vi "sub_log-load_ubx.vi"() -> ()   [LabVIEW 2019]
panel:
  in  "sel file - str":bool
  out "val":bool
  out "XY 그래프":cluster{"X":dbl, "Y":dbl}[](graph)
  in  "정지":bool
  out "heading imu":dbl[](array[numeric]) format="%01.1f"
  out "이전 부분 문자열":string
  out "heading tracing":dbl[](array[numeric]) format="%01.1f"
  out "latlong out":cluster{"Lat":dbl, "Long":dbl}[](array[cluster])
  out "tm out":cluster{"XE":dbl, "YN":dbl}[](array[cluster])
  out "n":i32=24061
  out "tm graph":cluster{"X":dbl, "Y":dbl}[](graph)=[{"X"=195463.43833256784, "Y"=532664.2368708845}, {"X"=195463.37935875848, "Y"=532664.3478879803}, {"X"=195463.37944915734, "Y"=532664.5143655398}, {"X"=195463.33526400154, "Y"=532664.6808671424}, {"X"=195463.23200460023, "Y"=532664.7734107748}, {"X"=195463.18778931902, "Y"=532664.8844198572}, {"X"=195463.158302417, "Y"=532664.939928406}, {"X"=195463.02545567148, "Y"=532664.9030055237}, {"X"=195462.96640151046, "Y"=532664.8660425695}, {"X"=195462.8335346741, "Y"=532664.7921246769}, {"X"=195462.74496347454, "Y"=532664.7551777533}, {"X"=195462.77457092013, "Y"=532664.9216392826}, {"X"=195463.42418674467, "Y"=532665.3652268056}, {"X"=195464.41330861498, "Y"=532665.9196151308}, {"X"=195465.49103164242, "Y"=532666.5664430471}, {"X"=195466.5393478853, "Y"=532667.4167596921}, {"X"=195467.73517878767, "Y"=532668.1375138587}, {"X"=195469.03423880192, "Y"=532668.7102321138}, {"X"=195470.27427462512, "Y"=532669.3014800847}, {"X"=195471.3814636429, "Y"=532669.8558052257}, {"X"=195472.53304832894, "Y"=532670.6320766001}, {"X"=195473.68450251664, "Y"=532671.1678805449}, {"X"=195474.82121809167, "Y"=532671.7406876583}, {"X"=195475.88423113854, "Y"=532672.4800124469}, {"X"=195476.94724399722, "Y"=532673.219337371}, {"X"=195478.0102466557, "Y"=532673.9401649248}, {"X"=195479.1764785589, "Y"=532674.5129566543}, {"X"=195480.32796180525, "Y"=532675.1042540387}, {"X"=195481.44992789478, "Y"=532675.6955675457}, {"X"=195482.6161893219, "Y"=532676.3238522782}, {"X"=195483.69397958953, "Y"=532677.1001650991}, {"X"=195484.6829887544, "Y"=532677.4510832544}, {"X"=195485.83431129332, "Y"=532677.7464212874}, {"X"=195487.10376165676, "Y"=532678.1526807427}, {"X"=195488.37312199303, "Y"=532678.3924628282}, {"X"=195489.36211083402, "Y"=532678.7063865255}, {"X"=195490.14448070675, "Y"=532679.0204218699}, {"X"=195491.16320601458, "Y"=532679.741275002}, {"X"=195492.19687926685, "Y"=532680.8135729311}, {"X"=195493.03851230364, "Y"=532681.5530193599}, {"X"=195494.1160914222, "Y"=532681.9408858792}, {"X"=195495.26754266868, "Y"=532682.4766928047}, {"X"=195496.15353049224, "Y"=532683.3640957345}, {"X"=195497.29010329436, "Y"=532683.6779408107}, {"X"=195498.39734841217, "Y"=532684.3432545831}, {"X"=195499.41604246455, "Y"=532685.0086162025}, {"X"=195500.8330559466, "Y"=532685.3778032307}, {"X"=195502.2500294698, "Y"=532685.6730004699}, {"X"=195503.38700991592, "Y"=532686.7452441752}, {"X"=195504.67135587469, "Y"=532687.4104634614}, {"X"=195505.88195899536, "Y"=532688.1682101777}, {"X"=195506.95982515637, "Y"=532689.0925060686}, {"X"=195508.05230036922, "Y"=532689.7393315544}, {"X"=195509.3218273631, "Y"=532690.2935744494}, {"X"=195510.63554014615, "Y"=532690.6813161802}, {"X"=195511.99361765472, "Y"=532691.2355118981}, {"X"=195513.08586370462, "Y"=532691.4568953742}, {"X"=195514.2076465018, "Y"=532691.7152581579}, {"X"=195515.32960795384, "Y"=532692.3065762268}, {"X"=195516.46638728245, "Y"=532693.0088715698}, {"X"=195517.58840795147, "Y"=532693.7111749877}, {"X"=195518.78410169733, "Y"=532694.1914688842}, {"X"=195519.99460336298, "Y"=532694.764242577}, {"X"=195521.1460511766, "Y"=532695.3000530777}, {"X"=195522.07599301488, "Y"=532695.5955147923}, {"X"=195523.1535293239, "Y"=532695.9093950319}, {"X"=195524.08341156298, "Y"=532696.0938719255}, {"X"=195524.5705894479, "Y"=532696.3710736269}, {"X"=195524.7034156071, "Y"=532696.3710024743}, {"X"=195524.74775044026, "Y"=532696.4819638014}, {"X"=195524.7478396172, "Y"=532696.6484413707}, {"X"=195524.85116866234, "Y"=532696.685381046}, {"X"=195524.89544404706, "Y"=532696.6853573297}, {"X"=195524.99875327287, "Y"=532696.6853019926}, {"X"=195525.07256539716, "Y"=532696.7222574817}, {"X"=195525.16117560753, "Y"=532696.8331950981}, {"X"=195525.29412064294, "Y"=532697.0550940447}, {"X"=195525.42702604536, "Y"=532697.2030029638}, {"X"=195525.57471962064, "Y"=532697.4063965041}, {"X"=195525.7075655717, "Y"=532697.4433203822}, {"X"=195525.79613614336, "Y"=532697.4802679741}, {"X"=195525.88469680815, "Y"=532697.4987180593}, {"X"=195525.98805555515, "Y"=532697.5911502724}, {"X"=195526.06185775693, "Y"=532697.609608263}, {"X"=195526.13568967706, "Y"=532697.683558776}, {"X"=195526.19477304455, "Y"=532697.776014701}, {"X"=195526.26859505233, "Y"=532697.8314677086}, {"X"=195526.3423873486, "Y"=532697.8314281941}, {"X"=195526.40143109093, "Y"=532697.849894091}, {"X"=195526.460474833, "Y"=532697.8683599874}, {"X"=195526.50474030682, "Y"=532697.8498387724}, {"X"=195526.4308588673, "Y"=532697.6834007172}, {"X"=195526.47517386338, "Y"=532697.7573670406}, {"X"=195526.50470068818, "Y"=532697.7758487416}, {"X"=195526.53420770136, "Y"=532697.7573354304}, {"X"=195526.54897606486, "Y"=532697.7758250341}, {"X"=195526.60804951593, "Y"=532697.8497834553}, {"X"=195526.68190123988, "Y"=532697.9607289893}, {"X"=195526.88855927964, "Y"=532698.0346083909}, {"X"=195526.96240109234, "Y"=532698.1270564198}, {"X"=195527.02141511615, "Y"=532698.0900297988}, {"X"=195527.08041924387, "Y"=532698.0345056687}, {"X"=195527.1247342301, "Y"=532698.108471994}, {"X"=195526.8884206263, "Y"=532697.7756432841}, {"X"=195526.77026381393, "Y"=532697.6092289329}, {"X"=195526.79978073458, "Y"=532697.6092131288}, {"X"=195526.8293570766, "Y"=532697.7201823699}, {"X"=195526.85892351624, "Y"=532697.8126541035}, {"X"=195527.00666656136, "Y"=532698.1085352066}, {"X"=195527.4348500131, "Y"=532698.4597587141}, {"X"=195528.24687212674, "Y"=532699.0327469374}, {"X"=195529.32456613673, "Y"=532699.6425880961}, {"X"=195530.63829630864, "Y"=532700.0673279922}, {"X"=195531.9963610663, "Y"=532700.6030294579}, {"X"=195533.33957819303, "Y"=532700.9722614696}, {"X"=195534.72692225696, "Y"=532701.0640074186}, {"X"=195536.1290939311, "Y"=532701.285228265}, {"X"=195537.44268517097, "Y"=532701.4510041233}, {"X"=195538.7415277862, "Y"=532701.6352855739}, {"X"=195540.0404394645, "Y"=532701.9490497827}, {"X"=195541.3246518252, "Y"=532702.3738071152}, {"X"=195542.65322822542, "Y"=532702.9650185935}, {"X"=195543.92269171606, "Y"=532703.4082817067}, {"X"=195545.19214520394, "Y"=532703.8330475076}, {"X"=195546.55014925377, "Y"=532704.2577662958}, {"X"=195547.87866584174, "Y"=532704.7379935593}, {"X"=195549.28095479903, "Y"=532705.181186705}, {"X"=195550.638899309, "Y"=532705.4949211149}, {"X"=195552.08545347524, "Y"=532705.9195936443}, {"X"=195553.48777154498, "Y"=532706.4182800212}, {"X"=195554.84590269416, "Y"=532707.0834677607}, {"X"=195556.0563803374, "Y"=532707.6192516707}, {"X"=195557.20781422194, "Y"=532708.1365696405}, {"X"=195558.40351345303, "Y"=532708.6353667225}, {"X"=195559.62873925007, "Y"=532709.1526457963}, {"X"=195560.85396489518, "Y"=532709.6699250496}, {"X"=195562.07921003803, "Y"=532710.2241994971}, {"X"=195563.289716231, "Y"=532710.8154769803}, {"X"=195564.54451719543, "Y"=532711.443726148}, {"X"=195565.81412549742, "Y"=532712.1644552109}, {"X"=195566.95081935, "Y"=532712.7187773762}, {"X"=195568.14656640016, "Y"=532713.3100633936}, {"X"=195569.38656895916, "Y"=532713.8643310885}, {"X"=195570.65612743786, "Y"=532714.4925733493}, {"X"=195571.82244535882, "Y"=532715.2503531169}, {"X"=195573.00352149023, "Y"=532716.0081252258}, {"X"=195574.12556370843, "Y"=532716.7659287783}, {"X"=195575.26236414464, "Y"=532717.5237246654}, {"X"=195576.51714361613, "Y"=532718.1149806204}, {"X"=195577.75707636445, "Y"=532718.5397670033}, {"X"=195579.0412646738, "Y"=532718.9275351231}, {"X"=195580.2369512657, "Y"=532719.4078378282}, {"X"=195581.55071486297, "Y"=532719.9065757681}, {"X"=195582.79060796814, "Y"=532720.2573728659}, {"X"=195583.9122771791, "Y"=532720.3122724262}, {"X"=195585.18163808706, "Y"=532720.570566735}, {"X"=195586.51004236046, "Y"=532720.8473275584}, {"X"=195587.80901763373, "Y"=532721.2905817559}, {"X"=195589.0932441141, "Y"=532721.7523414554}, {"X"=195590.28889067026, "Y"=532722.1586555662}, {"X"=195591.52884163495, "Y"=532722.620439012}, {"X"=195592.82786515707, "Y"=532723.1561815299}, {"X"=195594.12691777293, "Y"=532723.7474167764}, {"X"=195595.4554480201, "Y"=532724.264646632}, {"X"=195596.72497370603, "Y"=532724.837400335}, {"X"=195597.92078514092, "Y"=532725.5581731821}, {"X"=195599.1460547227, "Y"=532726.1679456017}, {"X"=195600.4893816471, "Y"=532726.759158516}, {"X"=195601.78835525474, "Y"=532727.2024148892}, {"X"=195603.01357563346, "Y"=532727.7197003352}, {"X"=195604.23879586247, "Y"=532728.2369859603}, {"X"=195605.5083106137, "Y"=532728.791243493}, {"X"=195606.777834921, "Y"=532729.3639987274}, {"X"=195608.06209800762, "Y"=532729.89975138}, {"X"=195609.3463609293, "Y"=532730.4355042303}, {"X"=195610.55678308988, "Y"=532730.8788085075}, {"X"=195611.8262484379, "Y"=532731.3405794604}, {"X"=195613.09573307371, "Y"=532731.8393456227}, {"X"=195614.30626164764, "Y"=532732.4861230355}, {"X"=195615.53155813567, "Y"=532733.1513903878}, {"X"=195616.8010810917, "Y"=532733.7241471487}, {"X"=195618.01163820943, "Y"=532734.4264176253}, {"X"=195619.25173131019, "Y"=532735.1656678186}, {"X"=195620.43281971622, "Y"=532735.9604416658}, {"X"=195621.56966180843, "Y"=532736.8107314138}, {"X"=195622.69168712775, "Y"=532737.5500439969}, {"X"=195623.8432193357, "Y"=532738.270843762}, {"X"=195624.9947416581, "Y"=532738.9731461777}, {"X"=195626.3085188666, "Y"=532739.5088861827}, {"X"=195627.50417074907, "Y"=532739.933703138}, {"X"=195628.75890443352, "Y"=532740.4509769174}, {"X"=195629.82173060603, "Y"=532740.8758637004}, {"X"=195630.91406376034, "Y"=532741.2822376763}, {"X"=195632.2130238219, "Y"=532741.7070012771}, {"X"=195633.55624922222, "Y"=532742.113244432}, {"X"=195635.03243521648, "Y"=532742.778383525}, {"X"=195636.36106617516, "Y"=532743.4990924905}, {"X"=195637.704397334, "Y"=532744.1088089084}, {"X"=195639.18054402331, "Y"=532744.6999587019}, {"X"=195640.62720270804, "Y"=532745.3466166832}, {"X"=195641.95580382948, "Y"=532746.0118340147}, {"X"=195643.31387325283, "Y"=532746.5845486206}, {"X"=195644.73091811733, "Y"=532747.046247619}, {"X"=195646.13317553644, "Y"=532747.4524620217}, {"X"=195647.47639933572, "Y"=532747.8587074166}, {"X"=195648.79020260356, "Y"=532748.4499434888}, {"X"=195650.08920879228, "Y"=532748.9671974168}, {"X"=195651.4619970308, "Y"=532749.4659156284}, {"X"=195652.89390520056, "Y"=532750.1310809287}, {"X"=195654.23720521078, "Y"=532750.6853074832}, {"X"=195655.60998330187, "Y"=532751.165528868}, {"X"=195656.95325412156, "Y"=532751.6642633328}, {"X"=195658.3260222799, "Y"=532752.1259876547}, {"X"=195659.68406075655, "Y"=532752.6432123989}, {"X"=195661.0568189934, "Y"=532753.0864396617}, {"X"=195662.38530200603, "Y"=532753.5296901399}, {"X"=195663.62526352247, "Y"=532754.0284793162}, {"X"=195664.9242295315, "Y"=532754.471745517}, {"X"=195666.41507324539, "Y"=532754.9519074148}, {"X"=195667.81734746048, "Y"=532755.3951204793}, {"X"=195669.1754711147, "Y"=532756.0788243498}, {"X"=195670.47450360752, "Y"=532756.6515739784}, {"X"=195671.7144545975, "Y"=532757.1318668477}, {"X"=195673.01350591303, "Y"=532757.741611891}, {"X"=195674.4453439012, "Y"=532758.2772983258}, {"X"=195675.8181195748, "Y"=532758.757523035}, {"X"=195677.24991892636, "Y"=532759.2192199171}, {"X"=195678.6965147357, "Y"=532759.7548994441}, {"X"=195680.1726461872, "Y"=532760.3275589806}, {"X"=195681.58975361122, "Y"=532760.918746801}, {"X"=195682.9478561166, "Y"=532761.565457895}, {"X"=195684.3059106409, "Y"=532762.1196816645}, {"X"=195685.73775670477, "Y"=532762.673867547}, {"X"=195687.0514976321, "Y"=532763.1541245902}, {"X"=195688.29143715004, "Y"=532763.6159224136}, {"X"=195689.51673271428, "Y"=532764.2996981493}, {"X"=195690.83054950094, "Y"=532764.9279358606}, {"X"=195692.2033899006, "Y"=532765.5376458303}, {"X"=195693.63525392523, "Y"=532766.1288280886}, {"X"=195695.06712727412, "Y"=532766.7385081005}, {"X"=195696.48426113735, "Y"=532767.3851909791}, {"X"=195697.9013566771, "Y"=532767.9578840624}, {"X"=195699.274138932, "Y"=532768.4566101402}, {"X"=195700.6174138786, "Y"=532768.9738491422}, {"X"=195701.84268861313, "Y"=532769.6206316698}, {"X"=195703.20075008267, "Y"=532770.1933560242}, {"X"=195704.4259768832, "Y"=532770.7476513837}, {"X"=195705.66599037888, "Y"=532771.3574318669}, {"X"=195707.0093024787, "Y"=532771.9486619369}, {"X"=195708.36731570578, "Y"=532772.4288995846}, {"X"=195709.65142314986, "Y"=532772.6872052341}, {"X"=195710.89134100443, "Y"=532773.1120113983}, {"X"=195712.21976121952, "Y"=532773.4442847518}, {"X"=195713.66621944733, "Y"=532773.721005208}, {"X"=195715.17156857622, "Y"=532773.720232995}, {"X"=195716.66205505346, "Y"=532773.5159960149}, {"X"=195718.06377359235, "Y"=532772.8863619665}, {"X"=195719.21443964881, "Y"=532771.9423990478}, {"X"=195720.37984534324, "Y"=532770.961433709}, {"X"=195721.42715623864, "Y"=532769.9250364729}, {"X"=195722.2234715443, "Y"=532768.6852952294}, {"X"=195722.81316091242, "Y"=532767.4271623343}, {"X"=195723.37340007036, "Y"=532766.2985271581}, {"X"=195723.8598003337, "Y"=532765.0774422467}, {"X"=195724.36091175413, "Y"=532763.7638622674}, {"X"=195724.96531281195, "Y"=532762.4132344332}, {"X"=195725.55501250137, "Y"=532761.1735992552}, {"X"=195726.14469344265, "Y"=532759.8969691027}, {"X"=195726.6163361366, "Y"=532758.675891914}, {"X"=195727.2504533032, "Y"=532757.7136968506}, {"X"=195727.92869433944, "Y"=532756.4555190526}, {"X"=195728.6955235518, "Y"=532755.2712860733}, {"X"=195729.27039029414, "Y"=532753.8836786455}, {"X"=195729.80093486852, "Y"=532752.403606346}, {"X"=195730.4347787353, "Y"=532750.9049837765}, {"X"=195730.5815966956, "Y"=532749.406610134}, {"X"=195731.171222524, "Y"=532748.0189953073}, {"X"=195731.90859293088, "Y"=532746.9457627758}, {"X"=195732.40967836019, "Y"=532745.5766907893}, {"X"=195732.9550674269, "Y"=532744.2630887484}, {"X"=195733.72191736553, "Y"=532743.1158512731}, {"X"=195734.4001888985, "Y"=532741.9131665553}, {"X"=195735.1226413439, "Y"=532740.5254842079}, {"X"=195735.88943527907, "Y"=532739.2672618876}, {"X"=195736.64145217667, "Y"=532737.9720521529}, {"X"=195737.27547769167, "Y"=532736.8248827985}, {"X"=195738.11613974278, "Y"=532735.7146031067}, {"X"=195738.85340834467, "Y"=532734.4378986182}, {"X"=195739.50221169676, "Y"=532733.3277169282}, {"X"=195740.10667400094, "Y"=532732.0880753087}, {"X"=195740.8586544795, "Y"=532730.7188759372}, {"X"=195741.40409299757, "Y"=532729.49776202}, {"X"=195741.84618512177, "Y"=532728.2027107645}, {"X"=195742.3768749644, "Y"=532727.0001019468}, {"X"=195742.9076215138, "Y"=532725.9084782144}, {"X"=195743.39398929762, "Y"=532724.6134044877}, {"X"=195744.013126419, "Y"=532723.207278077}, {"X"=195744.63225432741, "Y"=532721.7826542063}, {"X"=195745.3547855843, "Y"=532720.5429528507}, {"X"=195746.0919812887, "Y"=532719.118268969}, {"X"=195746.79966039592, "Y"=532717.6936001816}, {"X"=195747.24175398872, "Y"=532716.3985492358}, {"X"=195747.9051864799, "Y"=532715.0293956088}, {"X"=195748.46526311143, "Y"=532713.5678070722}, {"X"=195749.49760981172, "Y"=532712.1059782859}, {"X"=195750.293915986, "Y"=532710.8292448211}, {"X"=195751.04592827562, "Y"=532709.5155389357}, {"X"=195751.7389728836, "Y"=532708.3313456943}, {"X"=195752.29925753924, "Y"=532707.2767025982}, {"X"=195752.71192028275, "Y"=532706.1481445385}, {"X"=195753.25736213874, "Y"=532704.9270314455}, {"X"=195753.92084354223, "Y"=532703.6503658611}, {"X"=195754.30404618176, "Y"=532702.6328079345}, {"X"=195754.48040499454, "Y"=532701.171414843}, {"X"=195754.89309653037, "Y"=532700.0983494235}, {"X"=195755.52714623124, "Y"=532698.9881765428}, {"X"=195755.93978163204, "Y"=532697.8041261351}, {"X"=195756.57385043486, "Y"=532696.7309483497}, {"X"=195757.16371916333, "Y"=532695.8057731603}, {"X"=195757.3255268149, "Y"=532694.751332799}, {"X"=195757.72334785637, "Y"=532693.4563049399}, {"X"=195758.13587114145, "Y"=532692.0502845659}, {"X"=195758.79930736014, "Y"=532690.6811318584}, {"X"=195758.78403241967, "Y"=532689.6637764573}, {"X"=195759.240916004, "Y"=532688.4242112334}, {"X"=195759.69774339427, "Y"=532687.0736609943}, {"X"=195759.84460529315, "Y"=532685.6492780475}, {"X"=195759.41583947267, "Y"=532684.1326997027}, {"X"=195758.97240891086, "Y"=532682.8011039457}, {"X"=195758.14539840442, "Y"=532681.7471656362}, {"X"=195757.30375131758, "Y"=532680.9337024934}, {"X"=195756.21133188534, "Y"=532680.3608344682}, {"X"=195755.05985954026, "Y"=532679.7510015663}, {"X"=195753.93796042065, "Y"=532679.2521388625}, {"X"=195752.75706481075, "Y"=532678.8272963505}, {"X"=195751.66452250947, "Y"=532678.0139613304}, {"X"=195750.5573532222, "Y"=532677.4595990579}, {"X"=195749.52402331898, "Y"=532676.9976869228}, {"X"=195748.44622954918, "Y"=532676.1658473113}, {"X"=195747.36849205822, "Y"=532675.4449928794}, {"X"=195746.290810889, "Y"=532674.8351236291}, {"X"=195745.19833337844, "Y"=532674.1512720064}, {"X"=195744.16492739005, "Y"=532673.541380482}, {"X"=195743.02828712834, "Y"=532673.0795217791}, {"X"=195741.84728638385, "Y"=532672.4512082365}, {"X"=195740.69588734352, "Y"=532671.9893573737}, {"X"=195739.41162389636, "Y"=532671.453584379}, {"X"=195738.21576978508, "Y"=532670.6403038115}, {"X"=195737.0641909624, "Y"=532669.827000825}, {"X"=195735.92730434085, "Y"=532668.884207918}, {"X"=195734.71665323706, "Y"=532667.99694536}, {"X"=195733.38802823474, "Y"=532667.2947183395}, {"X"=195732.08897673475, "Y"=532666.7034614908}, {"X"=195730.8194609841, "Y"=532666.1491847765}, {"X"=195729.6238321926, "Y"=532665.7798455975}, {"X"=195728.4134731497, "Y"=532665.4660066579}, {"X"=195727.26204402428, "Y"=532664.9486651311}, {"X"=195725.99261284957, "Y"=532664.5608667078}, {"X"=195724.737940077, "Y"=532664.1730609236}, {"X"=195723.42425205032, "Y"=532663.8222805613}, {"X"=195721.99266624395, "Y"=532663.8045159772}, {"X"=195720.7382963556, "Y"=532664.008631001}, {"X"=195719.4247882052, "Y"=532664.0093038892}, {"X"=195718.1112136924, "Y"=532663.880494437}, {"X"=195716.85655941642, "Y"=532663.5296848536}, {"X"=195715.4542154872, "Y"=532662.9754785681}, {"X"=195714.09614693484, "Y"=532662.4212498091}, {"X"=195712.92992000942, "Y"=532661.8299278051}, {"X"=195711.79314350273, "Y"=532661.1091082669}, {"X"=195710.65640479152, "Y"=532660.4622789088}, {"X"=195709.46063179703, "Y"=532659.8154800249}, {"X"=195708.26486811935, "Y"=532659.1871788186}, {"X"=195706.9805911164, "Y"=532658.6329133086}, {"X"=195705.65209539948, "Y"=532658.1896557942}, {"X"=195704.26456542176, "Y"=532657.7464288456}, {"X"=195703.0098525606, "Y"=532657.2846363022}, {"X"=195701.7108544465, "Y"=532656.8043692198}, {"X"=195700.51517542722, "Y"=532656.3425466822}, {"X"=195699.3194105807, "Y"=532655.7142467571}, {"X"=195698.03512292422, "Y"=532655.1414851197}, {"X"=195696.75077792138, "Y"=532654.4577386423}, {"X"=195695.45170276545, "Y"=532653.8294924858}, {"X"=195694.15263694277, "Y"=532653.219744039}, {"X"=195692.92733502324, "Y"=532652.5544652317}, {"X"=195691.73155952425, "Y"=532651.9076688897}, {"X"=195690.49161316885, "Y"=532651.4643681268}, {"X"=195689.26644431343, "Y"=532651.0580549442}, {"X"=195688.1002713215, "Y"=532650.5777214466}, {"X"=195686.97835472776, "Y"=532650.0603702457}, {"X"=195685.67931636007, "Y"=532649.5061156364}, {"X"=195684.36556704534, "Y"=532649.0443563825}, {"X"=195683.06655701948, "Y"=532648.5455946978}, {"X"=195681.72317558818, "Y"=532647.8618810399}, {"X"=195680.21745947032, "Y"=532647.196749044}, {"X"=195678.69697499572, "Y"=532646.5131274458}, {"X"=195677.2208137773, "Y"=532645.9219707467}, {"X"=195675.77416945004, "Y"=532645.3307990311}, {"X"=195674.3423984007, "Y"=532644.9615899959}, {"X"=195672.95485498113, "Y"=532644.499870746}, {"X"=195671.59680934862, "Y"=532644.0011414224}, {"X"=195670.29773067127, "Y"=532643.3728991848}, {"X"=195668.96918262966, "Y"=532642.83715998}, {"X"=195667.6406152357, "Y"=532642.2644259746}, {"X"=195666.326787025, "Y"=532641.654689513}, {"X"=195665.0276308012, "Y"=532640.87846805}, {"X"=195663.64003818273, "Y"=532640.32426282}, {"X"=195662.3262381879, "Y"=532639.7700195067}, {"X"=195660.9238386092, "Y"=532639.1233348618}, {"X"=195659.55096554992, "Y"=532638.4951326232}, {"X"=195658.20757095923, "Y"=532637.7929252476}, {"X"=195656.80515149722, "Y"=532637.1092462835}, {"X"=195655.32895820634, "Y"=532636.462600942}, {"X"=195653.779029582, "Y"=532635.9269792836}, {"X"=195652.40633834526, "Y"=532635.650230827}, {"X"=195651.07782643987, "Y"=532635.188484495}, {"X"=195649.70493272858, "Y"=532634.5232888666}, {"X"=195648.30249275087, "Y"=532633.8026163208}, {"X"=195646.914878569, "Y"=532633.2114188608}, {"X"=195645.5863466897, "Y"=532632.7126783902}, {"X"=195644.2430464333, "Y"=532632.1954483205}, {"X"=195642.899765306, "Y"=532631.7152134788}, {"X"=195641.60073080176, "Y"=532631.1794632399}, {"X"=195640.2869375556, "Y"=532630.6437209033}, {"X"=195639.12069130508, "Y"=532630.0339117139}, {"X"=195637.85116379944, "Y"=532629.4796491468}, {"X"=195636.62590220332, "Y"=532628.906866143}, {"X"=195635.32687652478, "Y"=532628.3896143831}, {"X"=195633.9541351042, "Y"=532628.0203814362}, {"X"=195632.58136455325, "Y"=532627.595656197}, {"X"=195631.42993393028, "Y"=532627.0968254019}, {"X"=195630.3374988116, "Y"=532626.5239738682}, {"X"=195629.1712415813, "Y"=532625.8956685659}, {"X"=195627.88693483852, "Y"=532625.3044202244}, {"X"=195626.6468552614, "Y"=532624.6206613784}, {"X"=195625.4363120348, "Y"=532623.9738822693}, {"X"=195624.13723645333, "Y"=532623.3641447271}, {"X"=195622.7938945972, "Y"=532622.7729280898}, {"X"=195621.45060101955, "Y"=532622.2741991952}, {"X"=195620.15154427642, "Y"=532621.7014572844}, {"X"=195618.83770936087, "Y"=532621.0917283068}, {"X"=195617.68617029116, "Y"=532620.3894268518}, {"X"=195616.43138878574, "Y"=532619.816662296}, {"X"=195615.07334546503, "Y"=532619.3364396779}, {"X"=195613.8776271504, "Y"=532618.8191370377}, {"X"=195612.68193782834, "Y"=532618.3573270874}, {"X"=195611.39776478527, "Y"=532618.0250463588}, {"X"=195610.08405500065, "Y"=532617.655786326}, {"X"=195608.8588869878, "Y"=532617.2679824525}, {"X"=195607.58942360172, "Y"=532616.843207027}, {"X"=195606.364235896, "Y"=532616.4184085085}, {"X"=195605.0947430646, "Y"=532615.9381409462}, {"X"=195603.7661572725, "Y"=532615.3469196094}, {"X"=195602.52612292024, "Y"=532614.7556518759}, {"X"=195601.33038369365, "Y"=532614.2013560244}, {"X"=195600.14949058768, "Y"=532613.8135301189}, {"X"=195598.95403364376, "Y"=532613.7956622569}, {"X"=195597.96517770475, "Y"=532613.7406906884}, {"X"=195597.0500660527, "Y"=532613.593192821}, {"X"=195595.98753404556, "Y"=532613.760230436}, {"X"=195594.8808530445, "Y"=532614.1677590973}, {"X"=195593.9069800996, "Y"=532614.5382228445}, {"X"=195593.16912784666, "Y"=532614.6865920865}, {"X"=195592.8296701543, "Y"=532614.6682736343}, {"X"=195592.77065524724, "Y"=532614.7052997858}, {"X"=195592.7411185184, "Y"=532614.6683203462}, {"X"=195592.68207433814, "Y"=532614.6498539838}, {"X"=195592.66729621668, "Y"=532614.6128667602}, {"X"=195592.5934836698, "Y"=532614.5759106774}, {"X"=195592.53441021167, "Y"=532614.501951799}, {"X"=195592.4753465131, "Y"=532614.4464904262}, {"X"=195592.43103165913, "Y"=532614.3725237636}, {"X"=195592.3719582004, "Y"=532614.2985648863}, {"X"=195592.34240195114, "Y"=532614.224590439}, {"X"=195592.2980480622, "Y"=532614.0766337563}, {"X"=195592.2241964734, "Y"=532613.9656876568}, {"X"=195592.13563507324, "Y"=532613.94723687}, {"X"=195592.10609833896, "Y"=532613.910257433}, {"X"=195592.07658112506, "Y"=532613.9102730061}, {"X"=195592.04704439262, "Y"=532613.8732935688}, {"X"=195592.01750765767, "Y"=532613.8363141319}, {"X"=195592.00273928896, "Y"=532613.8178244133}, {"X"=195592.00271977021, "Y"=532613.7808294029}, {"X"=195592.00270025147, "Y"=532613.7438343933}, {"X"=195592.00270025147, "Y"=532613.7438343933}, {"X"=195592.0174491016, "Y"=532613.725329101}, {"X"=195592.01743934228, "Y"=532613.7068315962}, {"X"=195592.00267097334, "Y"=532613.6883418768}, {"X"=195591.98789284946, "Y"=532613.6513546549}, {"X"=195591.98788309004, "Y"=532613.6328571483}, {"X"=195591.98785381182, "Y"=532613.5773646337}, {"X"=195592.00258313896, "Y"=532613.5218643313}, {"X"=195592.01732223015, "Y"=532613.4848615346}, {"X"=195592.03207107855, "Y"=532613.4663562423}, {"X"=195592.03205155992, "Y"=532613.4293612314}, {"X"=195592.06154925926, "Y"=532613.3923506486}, {"X"=195592.0762883487, "Y"=532613.355347852}, {"X"=195592.0910274383, "Y"=532613.318345055}, {"X"=195592.10575676884, "Y"=532613.2628447529}, {"X"=195592.10573725053, "Y"=532613.2258497429}, {"X"=195592.10571773225, "Y"=532613.1888547324}, {"X"=195592.00232939524, "Y"=532613.0409291971}, {"X"=195591.98749271376, "Y"=532612.8929569435}, {"X"=195592.06126624122, "Y"=532612.8559230003}, {"X"=195592.04656618807, "Y"=532612.9669158172}, {"X"=195592.0023098765, "Y"=532613.0039341871}, {"X"=195592.01707824663, "Y"=532613.0224239061}, {"X"=195592.0318173365, "Y"=532612.985421109}, {"X"=195592.01704896858, "Y"=532612.9669313905}, {"X"=195591.95799501296, "Y"=532612.9299675284}, {"X"=195591.94324616605, "Y"=532612.9484728205}, {"X"=195591.9137387061, "Y"=532612.966985898}, {"X"=195591.89901913362, "Y"=532613.0409837047}, {"X"=195591.9284094811, "Y"=532612.8005005656}, {"X"=195591.85451883735, "Y"=532612.6155644489}, {"X"=195591.8692774466, "Y"=532612.615556662}, {"X"=195591.85452859706, "Y"=532612.6340619546}, {"X"=195591.810262527, "Y"=532612.6525828195}, {"X"=195591.8102722868, "Y"=532612.6710803256}, {"X"=195591.8250504177, "Y"=532612.7080675485}, {"X"=195591.82504065795, "Y"=532612.6895700429}, {"X"=195591.8103015662, "Y"=532612.7265728399}, {"X"=195591.8103210858, "Y"=532612.7635678502}, {"X"=195591.81034060539, "Y"=532612.8005628611}, {"X"=195591.8251382556, "Y"=532612.874545095}, {"X"=195591.78088194676, "Y"=532612.9115634656}, {"X"=195591.75132568963, "Y"=532612.8375890191}, {"X"=195591.6923693325, "Y"=532612.9856002091}, {"X"=195591.61859581008, "Y"=532613.0226341563}, {"X"=195591.42671437137, "Y"=532612.9857403841}, {"X"=195591.2790794785, "Y"=532612.8933307371}, {"X"=195591.2347548469, "Y"=532612.800866576}, {"X"=195591.22000599912, "Y"=532612.8193718698}, {"X"=195591.08706138024, "Y"=532612.5974719021}, {"X"=195590.34869156487, "Y"=532611.7654736221}, {"X"=195589.35942518603, "Y"=532610.9336078579}, {"X"=195588.17845291996, "Y"=532610.3978036054}, {"X"=195586.95310695004, "Y"=532609.6770478563}, {"X"=195585.71309988567, "Y"=532609.1412751358}, {"X"=195584.3255260493, "Y"=532608.64257561}, {"X"=195582.7312825008, "Y"=532608.0514980314}, {"X"=195581.18120696727, "Y"=532607.256924785}, {"X"=195579.61646060398, "Y"=532606.6288371806}, {"X"=195578.08118228934, "Y"=532605.9082467211}, {"X"=195576.60485006266, "Y"=532605.021147744}, {"X"=195575.2613451449, "Y"=532604.1339786832}, {"X"=195574.2127674942, "Y"=532602.7842158496}, {"X"=195573.03150885942, "Y"=532601.7119861029}, {"X"=195571.71736341997, "Y"=532600.5288418973}, {"X"=195570.56557238166, "Y"=532599.364109334}, {"X"=195569.51707184722, "Y"=532598.1623271359}, {"X"=195568.67539796303, "Y"=532597.3488830772}, {"X"=195567.64171442192, "Y"=532596.2580783184}, {"X"=195566.48991240672, "Y"=532595.0748488177}, {"X"=195565.44142056635, "Y"=532593.8915646428}, {"X"=195564.24548929388, "Y"=532592.9858215251}, {"X"=195563.0495675855, "Y"=532592.0985760847}, {"X"=195561.91262125585, "Y"=532591.1003144302}, {"X"=195560.83469942468, "Y"=532590.0835240588}, {"X"=195559.60927929927, "Y"=532589.2332898064}, {"X"=195558.11829168882, "Y"=532588.5496745085}, {"X"=195556.84858526246, "Y"=532587.6809666988}, {"X"=195555.56417895464, "Y"=532586.9232519577}, {"X"=195554.04371265956, "Y"=532586.3136431088}, {"X"=195552.4791769567, "Y"=532586.0925056969}, {"X"=195551.19477985732, "Y"=532585.3532891341}, {"X"=195549.9992891674, "Y"=532585.2799357616}, {"X"=195548.67072415628, "Y"=532584.744215719}, {"X"=195547.34207024888, "Y"=532584.0420183511}, {"X"=195545.9544603637, "Y"=532583.4878326969}, {"X"=195544.72916598598, "Y"=532582.8780681903}, {"X"=195543.4154575831, "Y"=532582.5273161563}, {"X"=195541.96881253138, "Y"=532581.9731626579}, {"X"=195540.62538908122, "Y"=532581.2524767293}, {"X"=195539.20821157153, "Y"=532580.6058204317}, {"X"=195538.14486647607, "Y"=532579.2560700462}, {"X"=195536.87528501518, "Y"=532578.6278328338}, {"X"=195535.3991511619, "Y"=532578.1291887554}, {"X"=195533.90835734206, "Y"=532577.8155278693}, {"X"=195532.5208840026, "Y"=532577.5203095112}, {"X"=195531.11848369395, "Y"=532576.9106417043}, {"X"=195529.84892114083, "Y"=532576.3194005704}, {"X"=195528.57945740456, "Y"=532575.9131346706}, {"X"=195527.25084001143, "Y"=532575.2849305178}, {"X"=195525.95179920626, "Y"=532574.7676957963}, {"X"=195524.52001931716, "Y"=532574.4170099638}, {"X"=195523.25034689318, "Y"=532573.6222972885}, {"X"=195521.90691056824, "Y"=532572.8831168716}, {"X"=195520.57833185772, "Y"=532572.3289037995}, {"X"=195519.23490501285, "Y"=532571.6082213176}, {"X"=195517.52297728043, "Y"=532571.7571196866}, {"X"=195516.09194107016, "Y"=532572.7937481003}, {"X"=195515.14815011327, "Y"=532574.2185628951}, {"X"=195514.44048834906, "Y"=532575.6247535137}, {"X"=195513.5115162647, "Y"=532577.1605456001}, {"X"=195512.62678079013, "Y"=532578.6223239948}, {"X"=195511.72727702395, "Y"=532580.0656129149}, {"X"=195510.65056025717, "Y"=532581.3055245483}, {"X"=195509.9281511286, "Y"=532582.7302209986}, {"X"=195509.14669766554, "Y"=532584.1364517433}, {"X"=195508.45386601886, "Y"=532585.6721174882}, {"X"=195507.746295867, "Y"=532587.2447862388}, {"X"=195507.23059839956, "Y"=532588.8358493836}, {"X"=195506.52297900195, "Y"=532590.3160307239}, {"X"=195505.87443424232, "Y"=532591.8701703899}, {"X"=195505.07821371916, "Y"=532593.2579119712}, {"X"=195504.296781967, "Y"=532594.7011382018}, {"X"=195503.54486776434, "Y"=532596.1443486259}, {"X"=195502.7930533857, "Y"=532597.7725341647}, {"X"=195502.20353447436, "Y"=532599.3081448543}, {"X"=195501.31875353132, "Y"=532600.677436977}, {"X"=195500.4043958474, "Y"=532601.9357600645}, {"X"=195499.6819603667, "Y"=532603.3049649347}, {"X"=195498.90045076306, "Y"=532604.6002116561}, {"X"=195498.31083338545, "Y"=532605.9508475862}, {"X"=195497.55889132252, "Y"=532607.3385660601}, {"X"=195496.7478951065, "Y"=532608.6893214115}, {"X"=195495.9812348243, "Y"=532610.1510380083}, {"X"=195495.2883080301, "Y"=532611.5017298587}, {"X"=195494.44775546243, "Y"=532612.7785113378}, {"X"=195493.7843962346, "Y"=532614.2216749283}, {"X"=195493.20956890192, "Y"=532615.6277957964}, {"X"=195492.8560708969, "Y"=532616.9413097474}, {"X"=195492.69441484427, "Y"=532618.2177251973}, {"X"=195492.37048412714, "Y"=532619.62371078}, {"X"=195491.98752911997, "Y"=532621.0482257342}, {"X"=195491.89978601434, "Y"=532622.5465714568}, {"X"=195491.60544265076, "Y"=532624.0820236888}, {"X"=195491.39960100822, "Y"=532625.5249406205}, {"X"=195490.9133363483, "Y"=532626.9495113901}, {"X"=195490.63373193637, "Y"=532628.4479606905}, {"X"=195490.14743762554, "Y"=532629.8170389946}, {"X"=195489.58744046267, "Y"=532631.3526347189}, {"X"=195488.8503006696, "Y"=532632.8143360895}, {"X"=195488.2016825962, "Y"=532634.2204971884}, {"X"=195487.6564346656, "Y"=532635.7375875761}, {"X"=195487.06688126508, "Y"=532637.1992094042}, {"X"=195486.5805780533, "Y"=532638.5497904298}, {"X"=195486.0352307626, "Y"=532639.8819058755}, {"X"=195485.63762915655, "Y"=532641.5099017089}, {"X"=195485.2105005992, "Y"=532643.1194160096}, {"X"=195484.5913310666, "Y"=532644.396078918}, {"X"=195483.70648780235, "Y"=532645.6358904657}, {"X"=195483.36793111885, "Y"=532647.2823520155}, {"X"=195483.22125566518, "Y"=532648.9657048674}, {"X"=195483.20728714686, "Y"=532650.4270158395}, {"X"=195483.2966984221, "Y"=532652.0177535054}, {"X"=195483.19414867222, "Y"=532653.4236198391}, {"X"=195483.16534163136, "Y"=532654.7369587494}, {"X"=195483.28418993053, "Y"=532656.1797004169}, {"X"=195483.41761672034, "Y"=532657.2894789957}, {"X"=195483.35922260216, "Y"=532658.4733513234}, {"X"=195483.13859471306, "Y"=532659.8607839957}, {"X"=195482.91775687571, "Y"=532660.8597690387}, {"X"=195482.8738413421, "Y"=532661.5257032139}, {"X"=195482.59397949537, "Y"=532662.5432176926}, {"X"=195481.5765018577, "Y"=532664.1345539491}, {"X"=195480.1454859443, "Y"=532665.1711886859}, {"X"=195478.72882848952, "Y"=532665.4679154156}, {"X"=195477.23812821423, "Y"=532665.3022446644}, {"X"=195475.79156319142, "Y"=532664.8775851093}, {"X"=195474.536788625, "Y"=532664.3233393318}, {"X"=195473.25246678415, "Y"=532663.7136172145}, {"X"=195471.89442232816, "Y"=532663.233417836}, {"X"=195470.47725337502, "Y"=532662.5867731243}, {"X"=195469.045375841, "Y"=532662.0326241923}, {"X"=195467.68719038466, "Y"=532661.2934604064}, {"X"=195466.2848796816, "Y"=532660.8317834674}, {"X"=195464.9710597313, "Y"=532660.2590736568}, {"X"=195463.56863821676, "Y"=532659.5939246013}, {"X"=195462.31387209284, "Y"=532659.0581781679}, {"X"=195461.35444720622, "Y"=532658.8367291786}, {"X"=195461.1921134429, "Y"=532658.8553148793}, {"X"=195461.20695236351, "Y"=532659.0032869143}, {"X"=195461.17754585168, "Y"=532659.2067755216}, {"X"=195461.17759609755, "Y"=532659.2992630547}, {"X"=195461.192334524, "Y"=532659.2622600235}, {"X"=195461.14809913983, "Y"=532659.3362741027}, {"X"=195461.16292801118, "Y"=532659.4657486308}, {"X"=195461.19251540853, "Y"=532659.5952151398}, {"X"=195461.20744476985, "Y"=532659.9096647339}, {"X"=195461.2075955065, "Y"=532660.1871273324}, {"X"=195461.2077160958, "Y"=532660.4090974107}, {"X"=195461.2077964887, "Y"=532660.5570774641}, {"X"=195461.17842012993, "Y"=532660.8160585919}, {"X"=195461.13429529392, "Y"=532661.0935452443}, {"X"=195461.10497923088, "Y"=532661.4635114124}, {"X"=195461.09034130024, "Y"=532661.6854895088}, {"X"=195461.09049204085, "Y"=532661.9629521096}, {"X"=195461.06115588627, "Y"=532662.2959232635}, {"X"=195461.04656820564, "Y"=532662.6103888944}, {"X"=195461.01718180516, "Y"=532662.8508725158}, {"X"=195460.98784565667, "Y"=532663.1838436713}, {"X"=195460.9142439995, "Y"=532663.5353363897}, {"X"=195460.85540086965, "Y"=532663.8868210906}, {"X"=195460.8555415683, "Y"=532664.1457861833}]
  out "str":string="$GNGGA,065308.00,3723.59854,N,12656.92439,E,1,12,0.78,40.9,M,18.5,M,,*74"
  out "latlong":cluster{"Lat":dbl, "Long":dbl} {"Lat" format="%.8f"; "Long" format="%.8f"}
  in  "path":path=path "C:/Users/WEGO/Documents/GitHub/Ycar/LabVIEW/GPS/logfile/nmea-anyang-beomgye.txt"
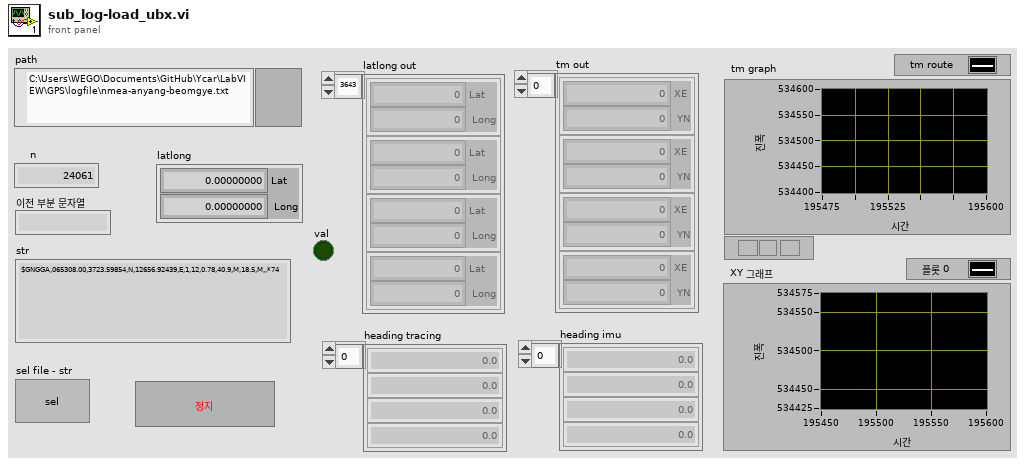
[diagram p1: front panel]
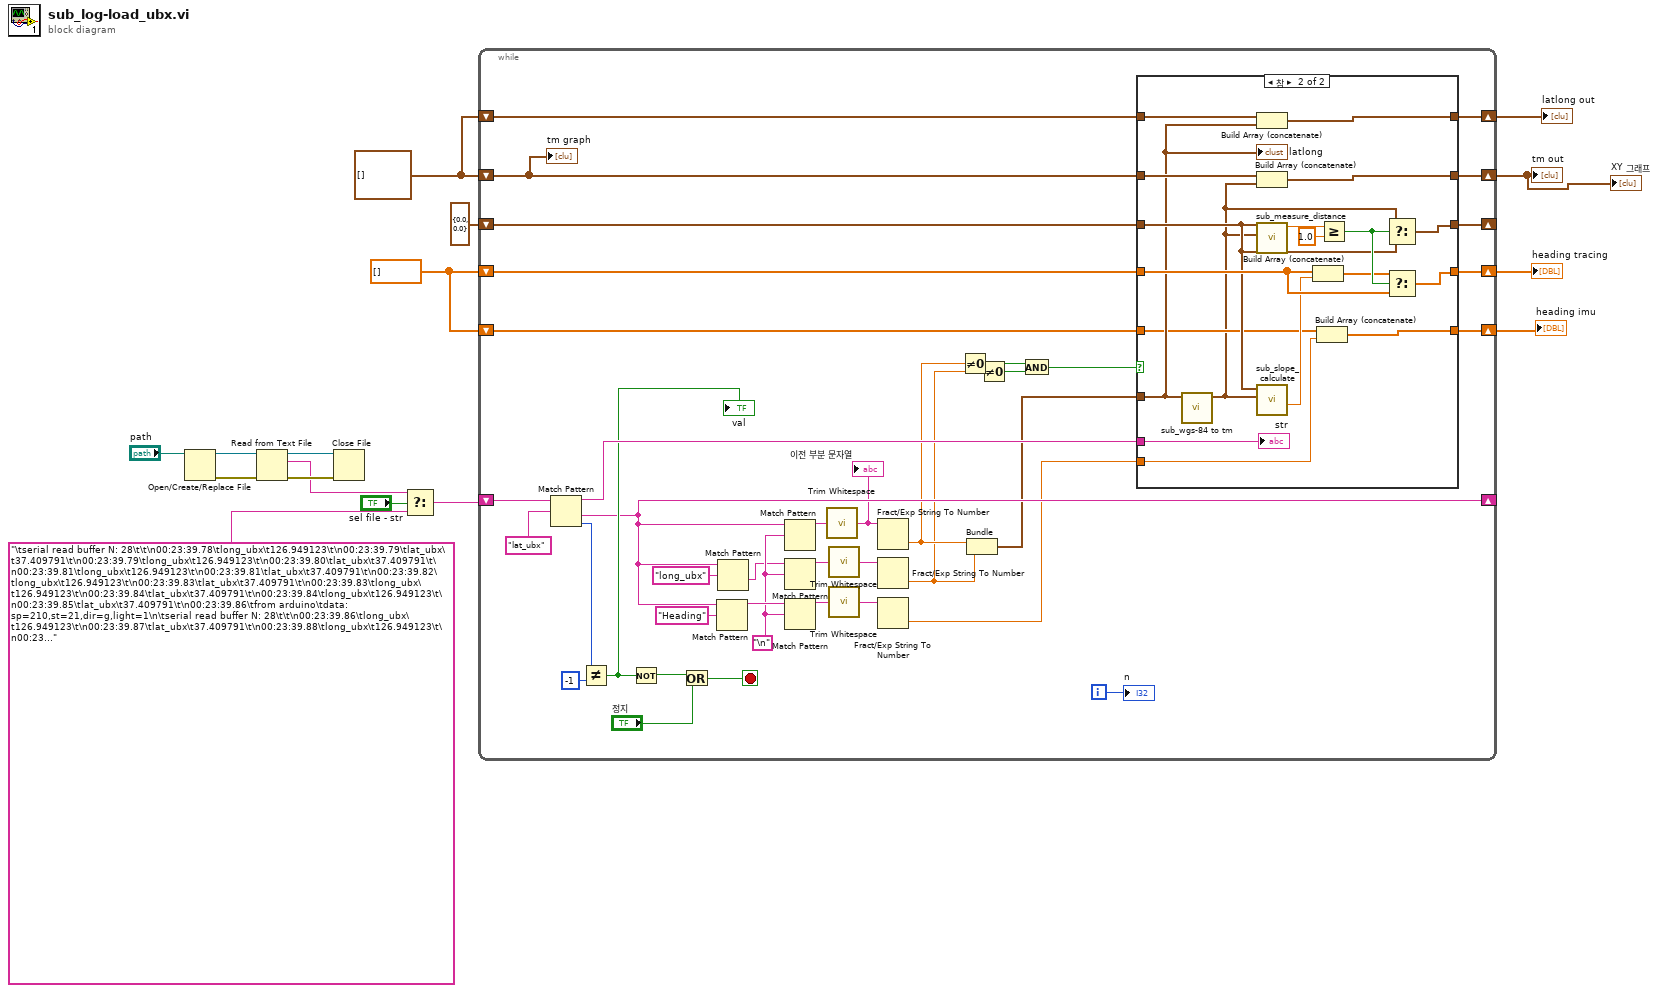
[diagram p0: block diagram]
diagram:
  w8 = dbl[] []
  w10 = cluster{"Lat":dbl, "Long":dbl}[] []
  n1 = Open/Create/Replace File(file path (use dialog)="path") -> (refnum out=w13:refnum<file>, error out=w16:errorcluster)  [unwired: 5 in, 1 out]
  n2 = Read from Text File(file (use dialog)=w13, error in=w16) -> (refnum out=w14:refnum<file>, text=w4:string, error out=w15:errorcluster)  [unwired: 2 in, 1 out]
  n3 = Close File(refnum=w14, error in=w15) -> ()  [unwired: 2 out]
  n4 = Select(t=w4, s="sel file - str", f="\tserial read buffer N: 28\t\t\n00:23:39.78\tlong_ubx\t126.949123\t\n00:23:39.79\tlat_ubx\t37.409791\t\n00:23:39.79\tlong_ubx\t126.949123\t\n00:23:39.80\tlat_ubx\t37.409791\t\n00:23:39.81\tlong_ubx\t126.949123\t\n00:23:39.81\tlat_ubx\t37.409791\t\n00:23:39.82\tlong_ubx\t126.949123\t\n00:23:39.83\tlat_ubx\t37.409791\t\n00:23:39.83\tlong_ubx\t126.949123\t\n00:23:39.84\tlat_ubx\t37.409791\t\n00:23:39.84\tlong_ubx\t126.949123\t\n00:23:39.85\tlat_ubx\t37.409791\t\n00:23:39.86\tfrom arduino\tdata: sp=210,st=21,dir=g,light=1\n\tserial read buffer N: 28\t\t\n00:23:39.86\tlong_ubx\t126.949123\t\n00:23:39.87\tlat_ubx\t37.409791\t\n00:23:39.88\tlong_ubx\t126.949123\t\n00:23:39.89\tlat_ubx\t37.409791\t\n00:23:39.90\tsysem resource usage: \tcpu: CPU Usage: 60 %\tmemory: 4382.3 MB\t\n00:23:39.90\tlong_ubx\t126.949123\t\n00:23:39.91\tlat_ubx\t37.409791\t\n00:23:39.92\tlong_ubx\t126.949123\t\n00:23:39.93\tfrom arduino\tdata: sp=210,st=21,dir=g,light=1\n\tserial read buffer N: 28\t\t\n00:23:39.94\tlat_ubx\t37.409791\t\n00:23:39.95\tlong_ubx\t126.949123\t\n00:23:39.96\tlat_ubx\t37.409791\t\n00:23:39.97\tlong_ubx\t126.949123\t\n00:23:39.98\tHeading\t226.560000\t\n00:23:39.98\timu-ang\t-0.130000\t-3.030000\t134.810000\n\t\n00:23:39.99\tlat_ubx\t37.409791\t\n00:23:40.00\tlong_ubx\t126.949123\t\n00:23:40.01\tlat_ubx\t37.409791\t\n00:23:40.02\tfrom arduino\tdata: sp=210,st=21,dir=g,light=1\n\tserial read buffer N: 28\t\t\n00:23:40.03\tlong_ubx\t126.949123\t\n00:23:40.03\tlat_ubx\t37.409791\t\n00:23:40.04\tublox gnss mode\t3D/DGNSS/FIXED\t\n00:23:40.05\tlong_ubx\t126.949123\t\n00:23:40.05\tlat_ubx\t37.409784\t\n00:23:40.06\tlong_ubx\t126.949121\t\n00:23:40.07\tlat_ubx\t37.409791\t\n00:23:40.08\tlong_ubx\t126.949123\t\n00:23:40.08\tlat_ubx\t37.409784\t\n00:23:40.09\tlong_ubx\t126.949121\t\n00:23:40.09\tfrom arduino\tdata: sp=210,st=21,dir=g,light=1\n\tserial read buffer N: 28\t\t\n00:23:40.10\tlat_ubx\t37.409784\t\n00:23:40.11\tlong_ubx\t126.949121\t\n00:23:40.11\tlat_ubx\t37.409784\t\n00:23:40.12\tlong_ubx\t126.949121\t\n00:23:40.12\tlat_ubx\t37.409784\t\n00:23:40.13\tlong_ubx\t126.949121\t\n00:23:40.14\tlat_ubx\t37.409784\t\n00:23:40.14\tlong_ubx\t126.949121\t\n00:23:40.15\tlat_ubx\t37.409784\t\n00:23:40.15\tlong_ubx\t126.949121\t\n00:23:40.16\tlat_ubx\t37.409784\t\n00:23:40.16\tlong_ubx\t126.949121\t\n00:23:40.17\tfrom arduino\tdata: sp=210,st=21,dir=g,light=1\n\tserial read buffer N: 28\t\t\n00:23:40.18\tlat_ubx\t37.409784\t\n00:23:40.18\tlong_ubx\t126.949121\t\n00:23:40.19\tlat_ubx\t37.409784\t\n00:23:40.19\tlong_ubx\t126.949121\t\n00:23:40.20\tlat_ubx\t37.409784\t\n00:23:40.21\tlong_ubx\t126.949121\t\n00:23:40.21\tlat_ubx\t37.409784\t\n00:23:40.22\tlong_ubx\t126.949121\t\n00:23:40.23\tlat_ubx\t37.409784\t\n00:23:40.24\tlong_ubx\t126.949121\t\n00:23:40.25\tHeading\t226.860000\t\n00:23:40.26\timu-ang\t-0.080000\t-3.050000\t134.510000\n\t\n00:23:40.27\tfrom arduino\tdata: sp=210,st=22,dir=g,light=1\n\tserial read buffer N: 28\t\t\n00:23:40.27\tlat_ubx\t37.409784\t\n00:23:40.28\tlong_ubx\t126.949121\t\n00:23:40.29\tlat_ubx\t37.409784\t\n00:23:40.30\tlong_ubx\t126.949121\t\n00:23:40.31\tlat_ubx\t37.409784\t\n00:23:40.31\tlong_ubx\t126.949121\t\n00:23:40.32\tlat_ubx\t37.409784\t\n00:23:40.33\tlong_ubx\t126.949121\t\n00:23:40.33\tfrom arduino\tdata: sp=210,st=22,dir=g,light=1\n\tserial read buffer N: 28\t\t\n00:23:40.34\tlat_ubx\t37.409784\t\n00:23:40.35\tlong_ubx\t126.949121\t\n00:23:40.35\tlat_ubx\t37.409784\t\n00:23:40.36\tlong_ubx\t126.949121\t\n00:23:40.37\tlat_ubx\t37.409784\t\n00:23:40.38\tlong_ubx\t126.949121\t\n00:23:40.39\tlat_ubx\t37.409784\t\n00:23:40.39\tlong_ubx\t126.949121\t\n00:23:40.40\tlat_ubx\t37.409784\t\n00:23:40.40\tlong_ubx\t126.949121\t\n00:23:40.41\tfrom arduino\tdata: sp=210,st=22,dir=g,light=1\n\tserial read buffer N: 28\t\t\n00:23:40.42\tlat_ubx\t37.409784\t\n00:23:40.42\tlong_ubx\t126.949121\t\n00:23:40.43\tlat_ubx\t37.409784\t\n00:23:40.43\tlong_ubx\t126.949121\t\n00:23:40.44\tlat_ubx\t37.409784\t\n00:23:40.45\tlong_ubx\t126.949121\t\n00:23:40.45\tlat_ubx\t37.409784\t\n00:23:40.46\tlong_ubx\t126.949121\t\n00:23:40.47\tlat_ubx\t37.409784\t\n00:23:40.47\tlong_ubx\t126.949121\t\n00:23:40.48\tlat_ubx\t37.409784\t\n00:23:40.49\tfrom arduino\tdata: sp=210,st=22,dir=g,light=1\n\tserial read buffer N: 28\t\t\n00:23:40.50\tlong_ubx\t126.949121\t\n00:23:40.51\tlat_ubx\t37.409784\t\n00:23:40.52\tlong_ubx\t126.949121\t\n00:23:40.53\tHeading\t226.960000\t\n00:23:40.53\timu-ang\t0.020000\t-3.070000\t134.410000\n\t\n00:23:40.54\tlat_ubx\t37.409784\t\n00:23:40.55\tlong_ubx\t126.949121\t\n00:23:40.56\tlat_ubx\t37.409784\t\n00:23:40.57\tlong_ubx\t126.949121\t\n00:23:40.57\tfrom arduino\tdata: sp=210,st=22,dir=g,light=1\n\tserial read buffer N: 28\t\t\n00:23:40.58\tlat_ubx\t37.409784\t\n00:23:40.59\tlong_ubx\t126.949121\t\n00:23:40.59\tlat_ubx\t37.409784\t\n00:23:40.60\tlong_ubx\t126.949121\t\n00:23:40.61\tlat_ubx\t37.409784\t\n00:23:40.61\tlong_ubx\t126.949121\t\n00:23:40.62\tlat_ubx\t37.409784\t\n00:23:40.63\tlong_ubx\t126.949121\t\n00:23:40.64\tlat_ubx\t37.409784\t\n00:23:40.64\tlong_ubx\t126.949121\t\n00:23:40.65\tfrom arduino\tdata: sp=210,st=22,dir=g,light=1\n\tserial read buffer N: 28\t\t\n00:23:40.66\tlat_ubx\t37.409784\t\n00:23:40.66\tlong_ubx\t126.949121\t\n00:23:40.67\tlat_ubx\t37.409784\t\n00:23:40.68\tlong_ubx\t126.949121\t\n00:23:40.68\tlat_ubx\t37.409784\t\n00:23:40.69\tlong_ubx\t126.949121\t\n00:23:40.70\tlat_ubx\t37.409784\t\n00:23:40.70\tlong_ubx\t126.949121\t\n00:23:40.71\tlat_ubx\t37.409784\t\n00:23:40.71\tlong_ubx\t126.949121\t\n00:23:40.72\tlat_ubx\t37.409784\t\n00:23:40.73\tlong_ubx\t126.949121\t\n00:23:40.73\tfrom arduino\tdata: sp=210,st=22,dir=g,light=1\n\tserial read buffer N: 28\t\t\n00:23:40.74\tlat_ubx\t37.409784\t\n00:23:40.74\tlong_ubx\t126.949121\t\n00:23:40.75\tlat_ubx\t37.409784\t\n00:23:40.76\tlong_ubx\t126.949121\t\n00:23:40.77\tlat_ubx\t37.409784\t\n00:23:40.78\tlong_ubx\t126.949121\t\n00:23:40.78\tlat_ubx\t37.409784\t\n00:23:40.79\tlong_ubx\t126.949121\t\n00:23:40.80\tHeading\t226.510000\t\n00:23:40.81\timu-ang\t-0.030000\t-3.420000\t134.860000\n\t\n00:23:40.82\tlat_ubx\t37.409784\t\n00:23:40.83\tfrom arduino\tdata: sp=210,st=22,dir=g,light=1\n\tserial read buffer N: 28\t\t\n00:23:40.84\tlong_ubx\t126.949121\t\n00:23:40.84\tlat_ubx\t37.409784\t\n00:23:40.85\tlong_ubx\t126.949121\t\n00:23:40.86\tlat_ubx\t37.409784\t\n00:23:40.87\tlong_ubx\t126.949121\t\n00:23:40.88\tlat_ubx\t37.409784\t\n00:23:40.89\tlong_ubx\t126.949121\t\n00:23:40.89\tfrom arduino\tdata: sp=210,st=21,dir=g,light=1\n\tserial read buffer N: 28\t\t\n00:23:40.90\tlat_ubx\t37.409784\t\n00:23:40.91\tsysem resource usage: \tcpu: CPU Usage: 62 %\tmemory: 4382.8 MB\t\n00:23:40.92\tlong_ubx\t126.949121\t\n00:23:40.92\tlat_ubx\t37.409784\t\n00:23:40.93\tlong_ubx\t126.949121\t\n00:23:40.93\tlat_ubx\t37.409784\t\n00:23:40.94\tlong_ubx\t126.949121\t\n00:23:40.95\tlat_ubx\t37.409784\t\n00:23:40.95\tlong_ubx\t126.949121\t\n00:23:40.96\tlat_ubx\t37.409784\t\n00:23:40.97\tlong_ubx\t126.949121\t\n00:23:40.97\tfrom arduino\tdata: sp=210,st=21,dir=g,light=1\n\tserial read buffer N: 28\t\t\n00:23:40.98\tlat_ubx\t37.409784\t\n00:23:40.98\tlong_ubx\t126.949121\t\n00:23:40.99\tlat_ubx\t37.409784\t\n00:23:41.00\tlong_ubx\t126.949121\t\n00:23:41.00\tlat_ubx\t37.409784\t\n00:23:41.01\tlong_ubx\t126.949121\t\n00:23:41.02\tlat_ubx\t37.409784\t\n00:23:41.02\tlong_ubx\t126.949121\t\n00:23:41.03\tlat_ubx\t37.409784\t\n00:23:41.04\tublox gnss mode\t3D/DGNSS/FIXED\t\n00:23:41.05\tlong_ubx\t126.949121\t\n00:23:41.06\tlat_ubx\t37.409776\t\n00:23:41.06\tfrom arduino\tdata: sp=210,st=21,dir=g,light=1\n\tserial read buffer N: 28\t\t\n00:23:41.07\tlong_ubx\t126.949120\t\n00:23:41.08\tlat_ubx\t37.409784\t\n00:23:41.10\tHeading\t225.680000\t\n00:23:41.10\timu-ang\t0.020000\t-3.160000\t135.690000\n\t\n00:23:41.11\tlong_ubx\t126.949121\t\n00:23:41.12\tlat_ubx\t37.409776\t\n00:23:41.13\tfrom arduino\tdata: sp=210,st=21,dir=g,light=1\n\tserial read buffer N: 28\t\t\n00:23:41.14\tlong_ubx\t126.949120\t\n00:23:41.14\tlat_ubx\t37.409776\t\n00:23:41.15\tlong_ubx\t126.949120\t\n00:23:41.16\tlat_ubx\t37.409776\t\n00:23:41.17\tlong_ubx\t126.949120\t\n00:23:41.17\tlat_ubx\t37.409776\t\n00:23:41.18\tlong_ubx\t126.949120\t\n00:23:41.19\tlat_ubx\t37.409776\t\n00:23:41.20\tlong_ubx\t126.949120\t\n00:23:41.20\tlat_ubx\t37.409776\t\n00:23:41.21\tlong_ubx\t126.949120\t\n00:23:41.21\tfrom arduino\tdata: sp=210,st=21,dir=g,light=1\n\tserial read buffer N: 28\t\t\n00:23:41.22\tlat_ubx\t37.409776\t\n00:23:41.23\tlong_ubx\t126.949120\t\n00:23:41.23\tlat_ubx\t37.409776\t\n00:23:41.24\tlong_ubx\t126.949120\t\n00:23:41.25\tlat_ubx\t37.409776\t\n00:23:41.25\tlong_ubx\t126.949120\t\n00:23:41.26\tlat_ubx\t37.409776\t\n00:23:41.26\tlong_ubx\t126.949120\t\n00:23:41.27\tlat_ubx\t37.409776\t\n00:23:41.27\tlong_ubx\t126.949120\t\n00:23:41.28\tlat_ubx\t37.409776\t\n00:23:41.29\tlong_ubx\t126.949120\t\n00:23:41.29\tfrom arduino\tdata: sp=210,st=21,dir=g,light=1\n\tserial read buffer N: 28\t\t\n00:23:41.30\tlat_ubx\t37.409776\t\n00:23:41.31\tlong_ubx\t126.949120\t\n00:23:41.31\tlat_ubx\t37.409776\t\n00:23:41.32\tlong_ubx\t126.949120\t\n00:23:41.32\tlat_ubx\t37.409776\t\n00:23:41.33\tlong_ubx\t126.949120\t\n00:23:41.34\tlat_ubx\t37.409776\t\n00:23:41.35\tlong_ubx\t126.949120\t\n00:23:41.36\tlat_ubx\t37.409776\t\n00:23:41.37\tlong_ubx\t126.949120\t\n00:23:41.37\tfrom arduino\tdata: sp=210,st=21,dir=g,light=1\n\tserial read buffer N: 28\t\t\n00:23:41.38\tlat_ubx\t37.409776\t\n00:23:41.39\tHeading\t224.960000\t\n00:23:41.40\timu-ang\t0.360000\t-3.140000\t136.410000\n\t\n00:23:41.41\tlong_ubx\t126.949120\t\n00:23:41.42\tlat_ubx\t37.409776\t\n00:23:41.42\tlong_ubx\t126.949120\t\n00:23:41.43\tlat_ubx\t37.409776\t\n00:23:41.44\tlong_ubx\t126.949120\t\n00:23:41.45\tlat_ubx\t37.409776\t\n00:23:41.45\tfrom arduino\tdata: sp=210,st=21,dir=g,light=1\n\tserial read buffer N: 28\t\t\n00:23:41.46\tlong_ubx\t126.949120\t\n00:23:41.47\tlat_ubx\t37.409776\t\n00:23:41.47\tlong_ubx\t126.949120\t\n00:23:41.48\tlat_ubx\t37.409776\t\n00:23:41.49\tlong_ubx\t126.949120\t\n00:23:41.50\tlat_ubx\t37.409776\t\n00:23:41.51\tlong_ubx\t126.949120\t\n00:23:41.52\tlat_ubx\t37.409776\t\n00:23:41.53\tlong_ubx\t126.949120\t\n00:23:41.53\tfrom arduino\tdata: sp=210,st=21,dir=g,light=1\n\tserial read buffer N: 28\t\t\n00:23:41.54\tlat_ubx\t37.409776\t\n00:23:41.54\tlong_ubx\t126.949120\t\n00:23:41.55\tlat_ubx\t37.409776\t\n00:23:41.56\tlong_ubx\t126.949120\t\n00:23:41.56\tlat_ubx\t37.409776\t\n00:23:41.57\tlong_ubx\t126.949120\t\n00:23:41.57\tlat_ubx\t37.409776\t\n00:23:41.58\tlong_ubx\t126.949120\t\n00:23:41.58\tlat_ubx\t37.409776\t\n00:23:41.59\tlong_ubx\t126.949120\t\n00:23:41.60\tlat_ubx\t37.409776\t\n00:23:41.60\tlong_ubx\t126.949120\t\n00:23:41.61\tfrom arduino\tdata: sp=210,st=21,dir=g,light=1\n\tserial read buffer N: 28\t\t\n00:23:41.62\tlat_ubx\t37.409776\t\n00:23:41.63\tlong_ubx\t126.949120\t\n00:23:41.64\tlat_ubx\t37.409776\t\n00:23:41.64\tlong_ubx\t126.949120\t\n00:23:41.65\tlat_ubx\t37.409776\t\n00:23:41.66\tlong_ubx\t126.949120\t\n00:23:41.67\tHeading\t224.430000\t\n00:23:41.68\timu-ang\t0.350000\t-2.730000\t136.940000\n\t\n00:23:41.69\tlat_ubx\t37.409776\t\n00:23:41.70\tfrom arduino\tdata: sp=210,st=21,dir=g,light=1\n\tserial read buffer N: 28\t\t\n00:23:41.70\tlong_ubx\t126.949120\t\n00:23:41.71\tlat_ubx\t37.409776\t\n00:23:41.72\tlong_ubx\t126.949120\t\n00:23:41.72\tlat_ubx\t37.409776\t\n00:23:41.73\tlong_ubx\t126.949120\t\n00:23:41.74\tlat_ubx\t37.409776\t\n00:23:41.75\tlong_ubx\t126.949120\t\n00:23:41.75\tlat_ubx\t37.409776\t\n00:23:41.76\tlong_ubx\t126.949120\t\n00:23:41.77\tfrom arduino\tdata: sp=210,st=20,dir=g,light=1\n\tserial read buffer N: 28\t\t\n00:23:41.78\tlat_ubx\t37.409776\t\n00:23:41.78\tlong_ubx\t126.949120\t\n00:23:41.79\tlat_ubx\t37.409776\t\n00:23:41.79\tlong_ubx\t126.949120\t\n00:23:41.80\tlat_ubx\t37.409776\t\n00:23:41.81\tlong_ubx\t126.949120\t\n00:23:41.81\tlat_ubx\t37.409776\t\n00:23:41.82\tlong_ubx\t126.949120\t\n00:23:41.82\tlat_ubx\t37.409776\t\n00:23:41.83\tlong_ubx\t126.949120\t\n00:23:41.84\tlat_ubx\t37.409776\t\n00:23:41.84\tlong_ubx\t126.949120\t\n00:23:41.85\tfrom arduino\tdata: sp=210,st=20,dir=g,light=1\n\tserial read buffer N: 28\t\t\n00:23:41.85\tlat_ubx\t37.409776\t\n00:23:41.86\tlong_ubx\t126.949120\t\n00:23:41.87\tlat_ubx\t37.409776\t\n00:23:41.88\tlong_ubx\t126.949120\t\n00:23:41.89\tlat_ubx\t37.409776\t\n00:23:41.89\tlong_ubx\t126.949120\t\n00:23:41.90\tlat_ubx\t37.409776\t\n00:23:41.91\tlong_ubx\t126.949120\t\n00:23:41.92\tsysem resource usage: \tcpu: CPU Usage: 64 %\tmemory: 4369.2 MB\t\n00:23:41.92\tHeading\t223.980000\t\n00:23:41.93\timu-ang\t0.430000\t-2.430000\t137.390000\n\t\n00:23:41.94\tlat_ubx\t37.409776\t\n00:23:41.95\tfrom arduino\tdata: sp=210,st=20,dir=g,light=1\n\tserial read buffer N: 28\t\t\n00:23:41.96\tlong_ubx\t126.949120\t\n00:23:41.96\tlat_ubx\t37.409776\t\n00:23:41.97\tlong_ubx\t126.949120\t\n00:23:41.98\tlat_ubx\t37.409776\t\n00:23:41.99\tlong_ubx\t126.949120\t\n00:23:41.99\tlat_ubx\t37.409776\t\n00:23:42.00\tlong_ubx\t126.949120\t\n00:23:42.01\tlat_ubx\t37.409776\t\n00:23:42.02\tfrom arduino\tdata: sp=210,st=20,dir=g,light=1\n\tserial read buffer N: 28\t\t\n00:23:42.02\tlong_ubx\t126.949120\t\n00:23:42.03\tlat_ubx\t37.409776\t\n00:23:42.04\tlong_ubx\t126.949120\t\n00:23:42.05\tlat_ubx\t37.409776\t\n00:23:42.05\tlong_ubx\t126.949120\t\n00:23:42.06\tlat_ubx\t37.409776\t\n00:23:42.06\tlong_ubx\t126.949120\t\n00:23:42.07\tlat_ubx\t37.409769\t\n00:23:42.08\tlong_ubx\t126.949119\t\n00:23:42.08\tlat_ubx\t37.409769\t\n00:23:42.09\tfrom arduino\tdata: sp=210,st=20,dir=g,light=1\n\tserial read buffer N: 28\t\t\n00:23:42.10\tlong_ubx\t126.949119\t\n00:23:42.10\tlat_ubx\t37.409769\t\n00:23:42.11\tlong_ubx\t126.949119\t\n00:23:42.11\tlat_ubx\t37.409769\t\n00:23:42.12\tlong_ubx\t126.949119\t\n00:23:42.13\tlat_ubx\t37.409769\t\n00:23:42.13\tlong_ubx\t126.949119\t\n00:23:42.14\tlat_ubx\t37.409769\t\n00:23:42.15\tlong_ubx\t126.949119\t\n00:23:42.16\tlat_ubx\t37.409769\t\n00:23:42.17\tlong_ubx\t126.949119\t\n00:23:42.17\tfrom arduino\tdata: sp=210,st=20,dir=g,light=1\n\tserial read buffer N: 28\t\t\n00:23:42.18\tlat_ubx\t37.409769\t\n00:23:42.19\tlong_ubx\t126.949119\t\n00:23:42.20\tHeading\t223.010000\t\n00:23:42.21\timu-ang\t0.630000\t-1.680000\t138.360000\n\t\n00:23:42.22\tlat_ubx\t37.409769\t\n00:23:42.23\tlong_ubx\t126.949119\t\n00:23:42.24\tlat_ubx\t37.409769\t\n00:23:42.24\tlong_ubx\t126.949119\t\n00:23:42.25\tfrom arduino\tdata: sp=210,st=20,dir=g,light=1\n\tserial read buffer N: 28\t\t\n00:23:42.26\tlat_ubx\t37.409769\t\n00:23:42.27\tlong_ubx\t126.949119\t\n00:23:42.28\tlat_ubx\t37.409769\t\n00:23:42.28\tlong_ubx\t126.949119\t\n00:23:42.29\tlat_ubx\t37.409769\t\n00:23:42.30\tlong_ubx\t126.949119\t\n00:23:42.30\tlat_ubx\t37.409769\t\n00:23:42.31\tlong_ubx\t126.949119\t\n00:23:42.32\tlat_ubx\t37.409769\t\n00:23:42.32\tlong_ubx\t126.949119\t\n00:23:42.33\tfrom arduino\tdata: sp=210,st=20,dir=g,light=1\n\tserial read buffer N: 28\t\t\n00:23:42.34\tlat_ubx\t37.409769\t\n00:23:42.34\tlong_ubx\t126.949119\t\n00:23:42.35\tlat_ubx\t37.409769\t\n00:23:42.36\tlong_ubx\t126.949119\t\n00:23:42.36\tlat_ubx\t37.409769\t\n00:23:42.37\tlong_ubx\t126.949119\t\n00:23:42.38\tlat_ubx\t37.409769\t\n00:23:42.38\tlong_ubx\t126.949119\t\n00:23:42.39\tlat_ubx\t37.409769\t\n00:23:42.39\tlong_ubx\t126.949119\t\n00:23:42.40\tlat_ubx\t37.409769\t\n00:23:42.41\tlong_ubx\t126.949119\t\n00:23:42.41\tfrom arduino\tdata: sp=210,st=20,dir=g,light=1\n\tserial read buffer N: 28\t\t\n00:23:42.42\tlat_ubx\t37.409769\t\n00:23:42.43\tlong_ubx\t126.949119\t\n00:23:42.44\tlat_ubx\t37.409769\t\n00:23:42.44\tlong_ubx\t126.949119\t\n00:23:42.45\tlat_ubx\t37.409769\t\n00:23:42.46\tlong_ubx\t126.949119\t\n00:23:42.48\tlat_ubx\t37.409769\t\n00:23:42.48\tHeading\t222.450000\t\n00:23:42.49\timu-ang\t0.500000\t-1.140000\t138.920000\n\t\n00:23:42.50\tlong_ubx\t126.949119\t\n00:23:42.51\tfrom arduino\tdata: sp=210,st=20,dir=g,light=1\n\tserial read buffer N: 28\t\t\n00:23:42.52\tlat_ubx\t37.409769\t\n00:23:42.53\tlong_ubx\t126.949119\t\n00:23:42.53\tlat_ubx\t37.409769\t\n00:23:42.54\tlong_ubx\t126.949119\t\n00:23:42.55\tlat_ubx\t37.409769\t\n00:23:42.56\tlong_ubx\t126.949119\t\n00:23:42.56\tlat_ubx\t37.409769\t\n00:23:42.57\tfrom arduino\tdata: sp=210,st=19,dir=g,light=1\n\tserial read buffer N: 28\t\t\n00:23:42.58\tlong_ubx\t126.949119\t\n00:23:42.59\tlat_ubx\t37.409769\t\n00:23:42.59\tlong_ubx\t126.949119\t\n00:23:42.60\tlat_ubx\t37.409769\t\n00:23:42.61\tlong_ubx\t126.949119\t\n00:23:42.61\tlat_ubx\t37.409769\t\n00:23:42.62\tlong_ubx\t126.949119\t\n00:23:42.63\tlat_ubx\t37.409769\t\n00:23:42.63\tlong_ubx\t126.949119\t\n00:23:42.64\tlat_ubx\t37.409769\t\n00:23:42.64\tlong_ubx\t126.949119\t\n00:23:42.65\tfrom arduino\tdata: sp=210,st=19,dir=g,light=1\n\tserial read buffer N: 28\t\t\n00:23:42.66\tlat_ubx\t37.409769\t\n00:23:42.66\tlong_ubx\t126.949119\t\n00:23:42.67\tlat_ubx\t37.409769\t\n00:23:42.68\tlong_ubx\t126.949119\t\n00:23:42.68\tlat_ubx\t37.409769\t\n00:23:42.69\tlong_ubx\t126.949119\t\n00:23:42.70\tlat_ubx\t37.409769\t\n00:23:42.70\tlong_ubx\t126.949119\t\n00:23:42.71\tlat_ubx\t37.409769\t\n00:23:42.71\tlong_ubx\t126.949119\t\n00:23:42.72\tlat_ubx\t37.409769\t\n00:23:42.73\tfrom arduino\tdata: sp=210,st=19,dir=g,light=1\n\tserial read buffer N: 28\t\t\n00:23:42.74\tlong_ubx\t126.949119\t\n00:23:42.75\tlat_ubx\t37.409769\t\n00:23:42.76\tlong_ubx\t126.949119\t\n00:23:42.77\tlat_ubx\t37.409769\t\n00:23:42.77\tHeading\t221.850000\t\n00:23:42.78\timu-ang\t0.530000\t-0.680000\t139.520000\n\t\n00:23:42.79\tlong_ubx\t126.949119\t\n00:23:42.80\tlat_ubx\t37.409769\t\n00:23:42.80\tlong_ubx\t126.949119\t\n00:23:42.81\tfrom arduino\tdata: sp=210,st=19,dir=g,light=1\n\tserial read buffer N: 28\t\t\n00:23:42.82\tlat_ubx\t37.409769\t\n00:23:42.82\tlong_ubx\t126.949119\t\n00:23:42.83\tlat_ubx\t37.409769\t\n00:23:42.84\tlong_ubx\t126.949119\t\n00:23:42.85\tlat_ubx\t37.409769\t\n00:23:42.85\tlong_ubx\t126.949119\t\n00:23:42.86\tlat_ubx\t37.409769\t\n00:23:42.87\tlong_ubx\t126.949119\t\n00:23:42.88\tlat_ubx\t37.409769\t\n00:23:42.89\tlong_ubx\t126.949119\t\n00:23:42.89\tfrom arduino\tdata: sp=210,st=19,dir=g,light=1\n\tserial read buffer N: 28\t\t\n00:23:42.90\tlat_ubx\t37.409769\t\n00:23:42.91\tlong_ubx\t126.949119\t\n00:23:42.91\tlat_ubx\t37.409769\t\n00:23:42.92\tlong_ubx\t126.949119\t\n00:23:42.92\tsysem resource usage: \tcpu: CPU Usage: 65 %\tmemory: 4366.6 MB\t\n00:23:42.93\tlat_ubx\t37.409769\t\n00:23:42.94\tlong_ubx\t126.949119\t\n00:23:42.94\tlat_ubx\t37.409769\t\n00:23:42.95\tlong_ubx\t126.949119\t\n00:23:42.95\tlat_ubx\t37.409769\t\n00:23:42.96\tlong_ubx\t126.949119\t\n00:23:42.97\tlat_ubx\t37.409769\t\n00:23:42.97\tfrom arduino\tdata: sp=210,st=19,dir=g,light=1\n\tserial read buffer N: 28\t\t\n00:23:42.98\tlong_ubx\t126.949119\t\n00:23:42.99\tlat_ubx\t37.409769\t\n00:23:43.00\tlong_ubx\t126.949119\t\n00:23:43.00\tlat_ubx\t37.409769\t\n00:23:43.01\tlong_ubx\t126.949119\t\n00:23:43.02\tlat_ubx\t37.409769\t\n00:23:43.02\tlong_ubx\t126.949119") -> (s? t:f=w2:string)
  n5 = while {
    shift-right: [w54] -> w6
    shift-left: w10 -> [w23]
    shift-right: [w37] -> _
    shift-left: w2 -> [w26]
    shift-right: [w50] -> w5
    shift-left: w10 -> [w24]
    shift-right: [w46] -> w11
    shift-left: w8 -> [w47]
    shift-right: [w48] -> _
    shift-left: cluster{"Y(E)":dbl, "X(N)":dbl} {"Y(E)"=0.0, "X(N)"=0.0} ("TM") -> [w49]
    shift-right: [w36] -> w7
    shift-left: w8 -> [w34]
    i -> [w53]
    stop <- w27 stop-if-true
    w33 = "\n"
    n6 = Match Pattern(string=w26, regular expression="lat_ubx" ("정규식")) -> (before substring=w51:string, after substring=w37:string, offset past match=w52:i32)  [unwired: 1 in, 1 out]
    n7 = Not Equal?(x=w52, y=-1) -> (x != y?=w41:bool)
    "val" <- w41
    n8 = Not(x=w41) -> (.not. x?=w29:bool)
    n9 = Or(x=w29, y="정지") -> (x .or. y?=w27:bool)
    n10 = Match Pattern(string=w37, regular expression="Heading" ("정규식")) -> (before substring=w39:string)  [unwired: 1 in, 3 out]
    n11 = Match Pattern(string=w37, regular expression="long_ubx" ("정규식")) -> (after substring=w25:string)  [unwired: 1 in, 3 out]
    n12 = Match Pattern(string=w37, regular expression=w33) -> (before substring=w43:string)  [unwired: 1 in, 3 out]
    n13 = Match Pattern(string=w25, regular expression=w33) -> (before substring=w42:string)  [unwired: 1 in, 3 out]
    n14 = Match Pattern(string=w39, regular expression=w33) -> (before substring=w40:string)  [unwired: 1 in, 3 out]
    n15 = call <vilib>:"Trim Whitespace.vi"("string"=w43) -> ("trimmed string"=w32:string)  [unwired: 1 in]
    "이전 부분 문자열" <- w32
    n16 = call <vilib>:"Trim Whitespace.vi"("string"=w42) -> ("trimmed string"=w31:string)  [unwired: 1 in]
    n17 = call <vilib>:"Trim Whitespace.vi"("string"=w40) -> ("trimmed string"=w30:string)  [unwired: 1 in]
    n18 = Fract/Exp String To Number(string=w32) -> (number=w20:dbl)  [unwired: 3 in, 1 out]
    n19 = Fract/Exp String To Number(string=w31) -> (number=w18:dbl)  [unwired: 3 in, 1 out]
    n20 = Fract/Exp String To Number(string=w30) -> (number=w35:dbl)  [unwired: 3 in, 1 out]
    n21 = Not Equal To 0?(x=w20) -> (x != 0?=w21:bool)
    n22 = Bundle(w20, w18) -> (w22:cluster{dbl, dbl})  [unwired: 1 in]
    n23 = Not Equal To 0?(x=w18) -> (x != 0?=w19:bool)
    n24 = And(x=w21, y=w19) -> (x .and. y?=w17:bool)
    n25 = case shown="참" w17 {
      tunnel: [w60 w79] -> w54
      tunnel: w23 -> [w60 w78]
      tunnel: w51 -> [_ w77]
      tunnel: w22 -> [_ w65]
      tunnel: [w59 w76] -> w50
      tunnel: w24 -> [w59 w75]
      tunnel: w49 -> [w58 w66]
      tunnel: [w58 w72] -> w48
      tunnel: w47 -> [w57 w68]
      tunnel: [w57 w69] -> w46
      tunnel: [w56 w64] -> w36
      tunnel: w35 -> [_ w63]
      tunnel: w34 -> [w56 w62]
      frame False {
      }
      frame True {
        n26 = call "sub_wgs-84 to tm.vi"("in_lon-lat"=w65) -> ("TM"=w61:cluster{"Y(E)":dbl, "X(N)":dbl})  [unwired: 10 in]
        n27 = Build Array (concatenate)(w75, w65) -> (w76:cluster{"Lat":dbl, "Long":dbl}[])
        n28 = Build Array (concatenate)(w78, w61) -> (w79:cluster{"Y(E)":dbl, "X(N)":dbl}[])
        n29 = call "sub_measure_distance.vi"("pt 2"=w61, "pt 1"=w66) -> ("distance"=w74:dbl)  [unwired: 9 in]
        n30 = call "sub_slope_calculate.vi"("point n+1"=w61, "point n"=w66) -> ("deg_gps-base"=w67:dbl)  [unwired: 7 in, 2 out]
        n31 = Build Array (concatenate)(w68, w67) -> (w70:dbl[])
        n32 = Build Array (concatenate)(w62, w63) -> (w64:dbl[])
        n33 = Greater Or Equal?(x=w74, y=1.0) -> (x >= y?=w71:bool)
        n34 = Select(t=w61, s=w71, f=w66) -> (s? t:f=w72:cluster{"Y(E)":dbl, "X(N)":dbl})
        n35 = Select(t=w70, s=w71, f=w68) -> (s? t:f=w69:dbl[])
        "str" <- w77
        "latlong" <- w65
      }
    }
    "n" <- w53
    "tm graph" <- w23
  }
  "tm out" <- w6
  "latlong out" <- w5
  "heading tracing" <- w11
  "heading imu" <- w7
  "XY 그래프" <- w6
